vi "RT Main.vi"() -> ()   [LabVIEW 2018]
uses:
  <vilib>/rvi/interface/nirviOpenFPGA/nirviOpenFPGA.xnode
  <vilib>/rvi/interface/nirviCloseFPGA/nirviCloseFPGA.xnode
  <vilib>/rvi/interface/nirviReadWriteControl/nirviReadWriteControl.xnode
  <vilib>/addons/control/pid/NI_PID_pid.lvlib
  <vilib>/rvi/interface/Simulation/niFpgaSimulationCallBeginRW.vi
  <vilib>/rvi/errors/niLvFpgaAdjustHostInterfaceError.vi
  FPGA Bitfiles/WattBalanceRev1_FPGATarget_FPGAMain_lNctXsg1hzM.lvbitx
  FPGA Main.vi
  <vilib>/addons/control/pid/pid.llb/PID (DBL).vi
  <vilib>/FPGAPlugInAG/Dynamic/niLvFpga_Close_Dynamic.vi
  Type Defs/Control Mode Type Def.ctl
panel:
  in  "Period (sec)":dbl
  in  "Control Mode":T1=enum."Manual"
  in  "Manual Voice Coil Voltage":dbl format="%.2f"
  in  "Voltage Limits":cluster{"Max Voltage":dbl, "Min Voltage":dbl}
  in  "PID":cluster{"Kp":dbl, "Ki":dbl, "Kd":dbl}
  in  "Set Point (µm)":dbl
  in  "Abort":bool
  in  "Amplifier On/Off":bool
  out "Displacement (µm)":dbl format="%#.2g"
  out "Voice Coil Voltage":dbl format="%.2f"
  out "Cap Probe Voltage Chart":dbl(graph) caption="Waveform Chart - dark"
  # "Sine Wave Controls"
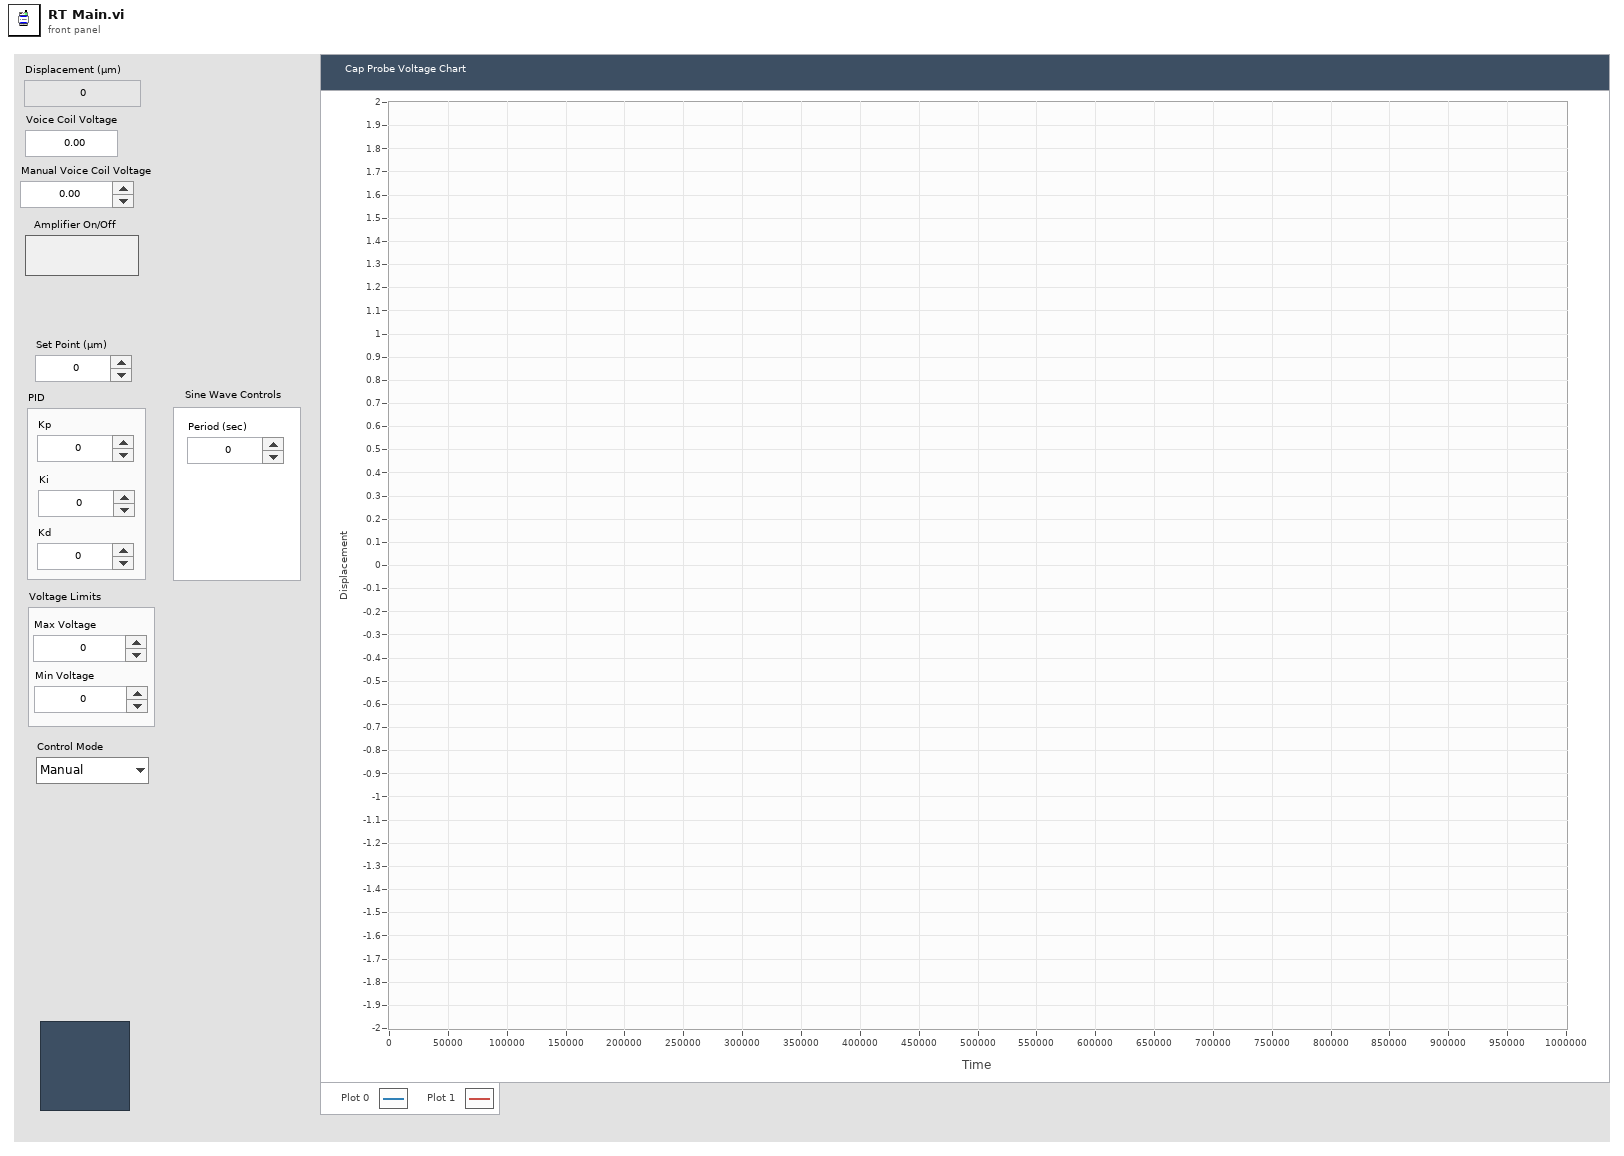
[diagram p1: front panel]
types:
  T1 = typedef "Control Mode Type Def.ctl" = enum16{"PID", "Manual"}
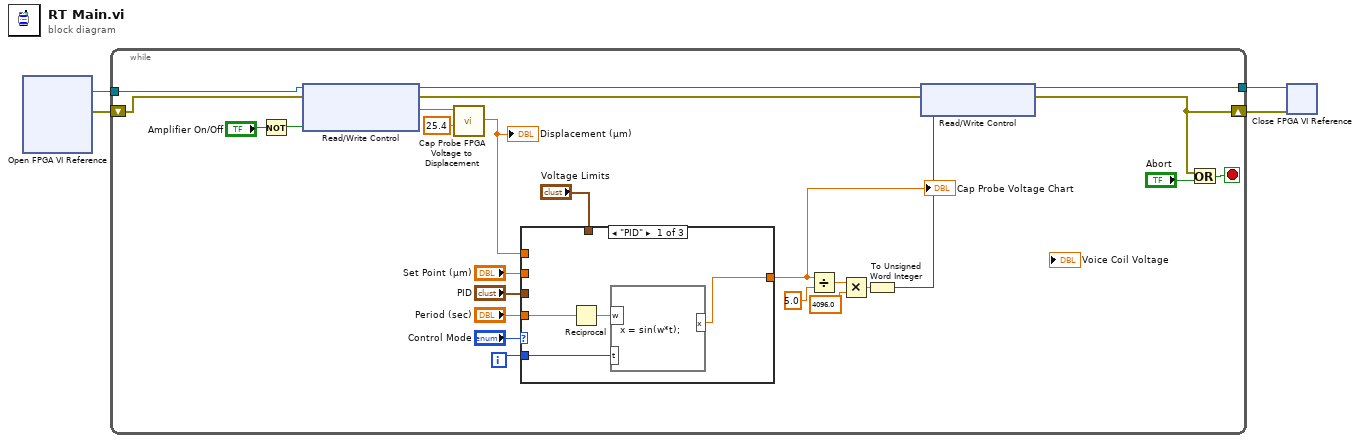
[diagram p0: block diagram]
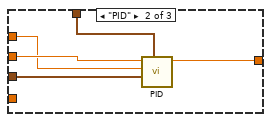
[diagram p2: hidden frame]
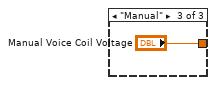
[diagram p3: hidden frame]
diagram:
  n1 = xnode "Open FPGA VI Reference"() -> ("FPGA VI Reference Out"=w4:refnum<k20>, "error out"=w3:errorcluster)  [unwired: 2 in]
  n2 = while {
    tunnel: w4 -> [w21]
    shift-right: [w7] -> w2
    shift-left: w3 -> [w18]
    tunnel: [w14] -> w1
    i -> [w9]
    stop <- w28 stop-if-true
    n3 = Not(x="Amplifier On/Off") -> (.not. x?=w19:bool)
    n4 = xnode "Read/Write Control"("FPGA VI Reference In"=w21, "error in"=w18, "Amplifier On/Off"=w19) -> ("FPGA VI Reference Out"=w15:refnum<k20>, "error out"=w13:errorcluster, "Cap Probe Voltage"=w20)
    n5 = call "Cap Probe FPGA Voltage to Displacement.vi"("Micrometers per Volt"=25.4, "Cap Probe FPGA Voltage"=w20) -> ("Cap Probe Displacement"=w6:dbl)  [unwired: 9 in]
    "Displacement (µm)" <- w6
    n6 = case shown="\"PID\"" "Control Mode" {
      tunnel: "Set Point (µm)" -> [_ w38 _]
      tunnel: w6 -> [_ w37 _]
      tunnel: "PID" -> [_ w36 _]
      tunnel: "Voltage Limits" -> [_ w35 _]
      tunnel: [w30 w34 "Manual Voice Coil Voltage"] -> w5
      tunnel: "Period (sec)" -> [w32 _ _]
      tunnel: w9 -> [w31 _ _]
      frame "PID" {
        n7 = Reciprocal(x=w32) -> (1/x=w33:dbl)
        n8 = formula code="x = sin(w*t);"("w"=w33, "t"=w31) -> ("x"=w30:dbl)
      }
      frame "PID" {
        n9 = call-poly <vilib>:"PID.vi"("output range"=w35, "PID gains"=w36, "process variable"=w37, "setpoint"=w38) -> ("output"=w34:dbl)  [unwired: 6 in, 1 out]
      }
      frame "Manual" {
      }
    }
    "Cap Probe Voltage Chart" <- w5
    n10 = Divide(x=w5, y=5.0) -> (x/y=w24:dbl)
    n11 = Multiply(x=w24, y=4096.0) -> (x*y=w22:dbl)
    n12 = To Unsigned Word Integer(number=w22) -> (unsigned 16bit integer=w12:u16)
    n13 = xnode "Read/Write Control"("FPGA VI Reference In"=w15, "error in"=w13, "Voice Coil Voltage"=w12) -> ("FPGA VI Reference Out"=w14:refnum<k20>, "error out"=w7:errorcluster)
    n14 = Or(x=w7, y="Abort") -> (x .or. y?=w28:bool)
  }
  n15 = xnode "Close FPGA VI Reference"("FPGA VI Reference In"=w1, "error in"=w2) -> ()  [unwired: 1 out]
